vi "Property Node Write Core.vi"(8 "error in (no error)":errorcluster, 9 "value":variant, 10 "property":string, 11 "SLSC Remote in":refnum<class "SLSC Remote.lvclass">) -> (0 "error out":errorcluster, 3 "SLSC Remote out":refnum<class "SLSC Remote.lvclass">)   [LabVIEW 2015, in "SLSC Remote.lvclass"]
uses:
  SLSC Remote.lvclass
  <vilib>/NI/i3 JSON/JSON Generation/Create Value Files/Create Value - Object.vi
  <vilib>/NI/i3 JSON/JSON Generation/Add Object Parameter Files/Add Object Parameter - String.vi
  <vilib>/NI/i3 JSON/JSON Generation/Add Object Parameter Files/Add Object Parameter - Known Type.vi
  <vilib>/NI/NI JSONRPC Server Framework/Classes/Server/Format Client Request (Auto-Increment).vi
  <vilib>/httpClient/POSTBuffer.vi
  <vilib>/NI/NI JSONRPC Server Framework/Classes/Server/JSONRPC Server.lvclass
  <vilib>/NI/i3 JSON/i3-json.lvlib
  <vilib>/httpClient/LabVIEWHTTPClient.lvlib
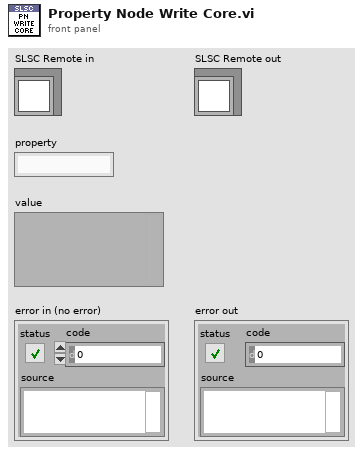
[diagram p1: front panel]
types:
  T1 = typedef "LabVIEWHTTPClient.lvlib/ClientHandle.ctl" = refnum<k1>
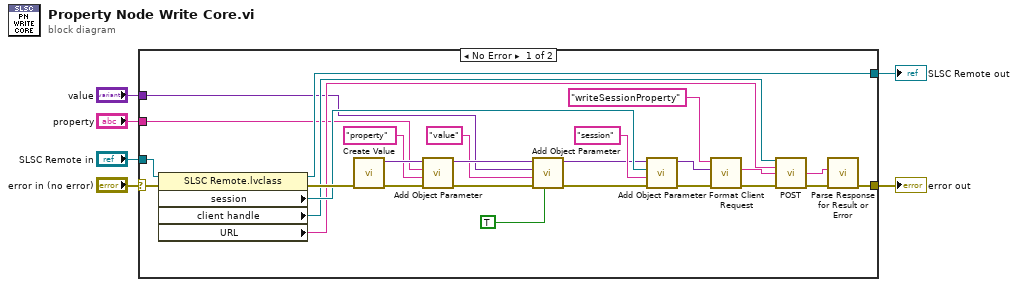
[diagram p0: block diagram]
diagram:
  n1 = case shown="No Error" "error in (no error)" {
    selector: "error in (no error)" -> [w29 w34]
    tunnel: "SLSC Remote in" -> [w32 w35]
    tunnel: [w31 w35] -> w3
    tunnel: [w15 w34] -> w4
    tunnel: "property" -> [w14 _]
    tunnel: "value" -> [w7 _]
    frame No Error {
      n2 = property class="SLSC Remote.lvclass"(reference=w32, error in=w29) -> (reference out=w31:refnum<class "SLSC Remote.lvclass">, error out=w28:errorcluster, "session"=w24:refnum<k21>, "client handle"=w20:T1, "URL"=w19:string)
      n3 = call-poly <vilib>:"Create Value.vi"("error in (no error)"=w28) -> ("error out"=w27:errorcluster, "JSON Tree"=w33:variant)  [unwired: 9 in]
      n4 = call-poly <vilib>:"Add Object Parameter.vi"("error in (no error)"=w27, "Name"="property", "String"=w14, "JSON Tree in (JSON Object)"=w33) -> ("error out"=w10:errorcluster, "JSON Tree out (JSON Object)"=w13:variant)  [unwired: 6 in]
      n5 = call-poly <vilib>:"Add Object Parameter.vi"("Add Parameter as JSON Tree?"=TRUE, "error in (no error)"=w10, "Name"="value", "Value"=w7, "JSON Tree in (JSON Object)"=w13) -> ("error out"=w11:errorcluster, "JSON Tree out (JSON Object)"=w12:variant)  [unwired: 5 in]
      n6 = call-poly <vilib>:"Add Object Parameter.vi"("error in (no error)"=w11, "Name"="session", "String"=w24, "JSON Tree in (JSON Object)"=w12) -> ("error out"=w21:errorcluster, "JSON Tree out (JSON Object)"=w22:variant)  [unwired: 6 in]
      n7 = call-poly <vilib>:"Format Client Request.vi"("error in (no error)"=w21, "params"=w22, "method"="writeSessionProperty") -> ("error out"=w18:errorcluster, "Request String"=w25:string)  [unwired: 7 in]
      n8 = call-poly <vilib>:"POST.vi"("client handle"=w20, "url"=w19, "buffer"=w25, "error in (no error)"=w18) -> ("body"=w17:string, "error out"=w16:errorcluster)  [unwired: 8 in, 2 out]
      n9 = call <vilib>:"Parse Response for Result or Error.vi"("error in"=w16, "Response String In"=w17) -> ("error out"=w15:errorcluster)  [unwired: 8 in, 1 out]
    }
    frame Error {
    }
  }
  "error out" <- w4
  "SLSC Remote out" <- w3
